vi "Format_text_fields.vi"(2 "error out":errorcluster, 3 "output cluster":T1, 4 "report out 2":refnum<class "NI_report.lvclass">) -> (0 "error out 2":errorcluster, 1 "report out":refnum<class "NI_report.lvclass">)   [LabVIEW 2010]
uses:
  <vilib>/Utility/NIReport.llb/NI_report.lvclass
  <vilib>/Utility/NIReport.llb/Append Report Text (str wrap).vi
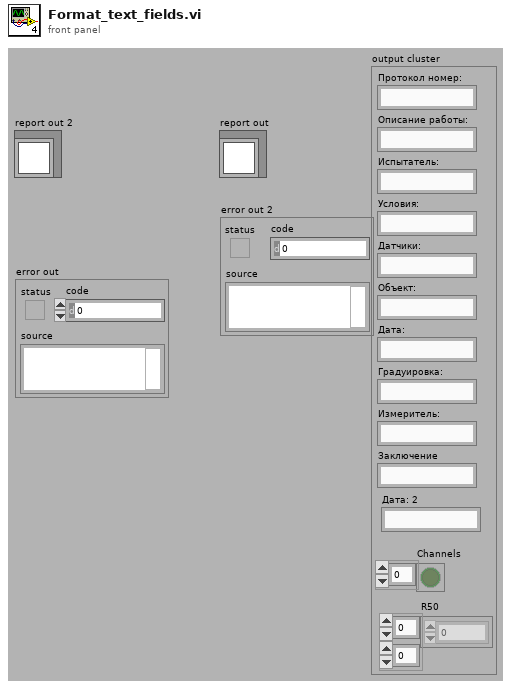
[diagram p1: front panel]
types:
  T1 = cluster{"Протокол номер:":string, "Описание работы:":string, "Испытатель:":string, "Условия:":string, "Датчики:":string, "Объект:":string, "Дата:":string, "Градуировка:":string, "Измеритель:":string, "Заключение":string, "Дата: 2":string, "Channels":bool[], "R50":dbl[][]}
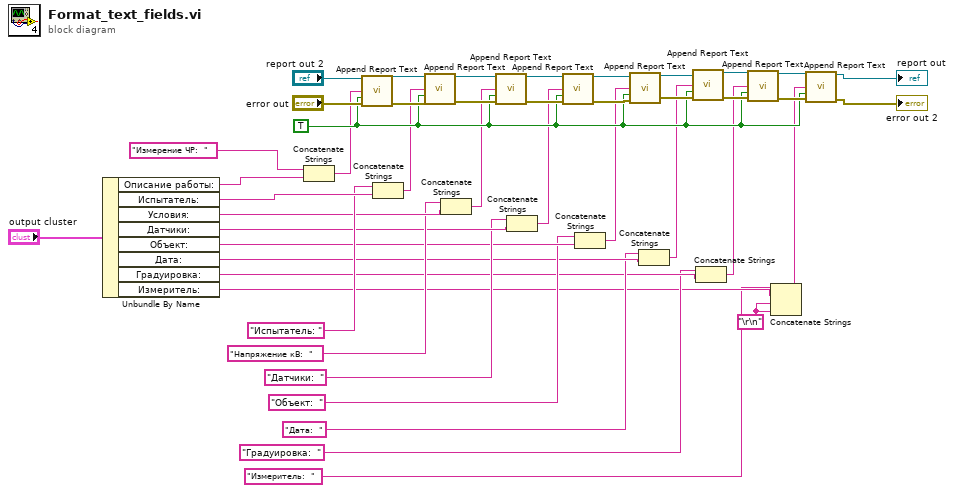
[diagram p0: block diagram]
diagram:
  w1 = "\r\n"
  w28 = TRUE ("append on new line? (F)")
  n1 = Unbundle By Name("output cluster") -> ("Описание работы:"=w25:string, "Испытатель:"=w22:string, "Условия:"=w19:string, "Датчики:"=w16:string, "Объект:"=w13:string, "Дата:"=w10:string, "Градуировка:"=w7:string, "Измеритель:"=w4:string)
  n2 = Concatenate Strings("Измерение ЧР:  " ("string"), w25) -> (w24:string)
  n3 = call-poly <vilib>:"Append Report Text.vi"("report in"="report out 2", "text"=w24, "append on new line? (F)"=w28, "error in (no error)"="error out") -> ("report out"=w41:refnum<class "NI_report.lvclass">, "error out"=w42:errorcluster)  [unwired: 2 in, 8 out]
  n4 = Concatenate Strings("Испытатель: " ("string"), w22) -> (w21:string)
  n5 = call-poly <vilib>:"Append Report Text.vi"("report in"=w41, "text"=w21, "append on new line? (F)"=w28, "error in (no error)"=w42) -> ("report out"=w39:refnum<class "NI_report.lvclass">, "error out"=w40:errorcluster)  [unwired: 2 in, 8 out]
  n6 = Concatenate Strings("Напряжение кВ:  " ("string"), w19) -> (w18:string)
  n7 = call-poly <vilib>:"Append Report Text.vi"("report in"=w39, "text"=w18, "append on new line? (F)"=w28, "error in (no error)"=w40) -> ("report out"=w37:refnum<class "NI_report.lvclass">, "error out"=w38:errorcluster)  [unwired: 2 in, 8 out]
  n8 = Concatenate Strings("Датчики:  " ("string"), w16) -> (w15:string)
  n9 = call-poly <vilib>:"Append Report Text.vi"("report in"=w37, "text"=w15, "append on new line? (F)"=w28, "error in (no error)"=w38) -> ("report out"=w35:refnum<class "NI_report.lvclass">, "error out"=w36:errorcluster)  [unwired: 2 in, 8 out]
  n10 = Concatenate Strings("Объект:  " ("string"), w13) -> (w12:string)
  n11 = call-poly <vilib>:"Append Report Text.vi"("report in"=w35, "text"=w12, "append on new line? (F)"=w28, "error in (no error)"=w36) -> ("report out"=w33:refnum<class "NI_report.lvclass">, "error out"=w34:errorcluster)  [unwired: 2 in, 8 out]
  n12 = Concatenate Strings("Дата:  " ("string"), w10) -> (w8:string)
  n13 = call-poly <vilib>:"Append Report Text.vi"("report in"=w33, "text"=w8, "append on new line? (F)"=w28, "error in (no error)"=w34) -> ("report out"=w32:refnum<class "NI_report.lvclass">, "error out"=w31:errorcluster)  [unwired: 2 in, 8 out]
  n14 = Concatenate Strings("Градуировка:  " ("string"), w7) -> (w5:string)
  n15 = call-poly <vilib>:"Append Report Text.vi"("report in"=w32, "text"=w5, "append on new line? (F)"=w28, "error in (no error)"=w31) -> ("report out"=w30:refnum<class "NI_report.lvclass">, "error out"=w29:errorcluster)  [unwired: 2 in, 8 out]
  n16 = Concatenate Strings("Измеритель:  " ("string"), w4, w1, w1) -> (w3:string)
  n17 = call-poly <vilib>:"Append Report Text.vi"("report in"=w30, "text"=w3, "append on new line? (F)"=w28, "error in (no error)"=w29) -> ("report out"=→"report out":refnum<class "NI_report.lvclass">, "error out"=→"error out 2":errorcluster)  [unwired: 2 in, 8 out]
